vi "MAVLink Packet Sequence.vi"(7 "FGV Method":T1, 11 "Packet Sequence In":u8) -> (3 "Packet Sequence Out":u8)   [LabVIEW 2014]
uses:
  Controls/FGV Methods.ctl
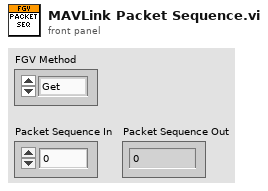
[diagram p1: front panel]
types:
  T1 = typedef "FGV Methods.ctl" = enum16{"Get", "Set"}
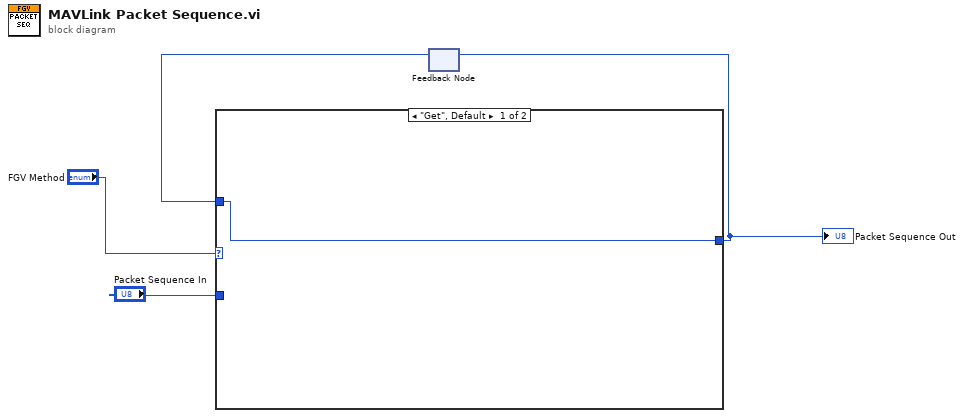
[diagram p0: block diagram]
diagram:
  n1 = feedback #1() -> (w3:u8)  [unwired: 1 in]
  n2 = case shown="\"Get\", Default" "FGV Method" {
    tunnel: "Packet Sequence In" -> [_ w6]
    tunnel: [w5 w6] -> w1
    tunnel: w3 -> [w5 _]
    frame "Get", Default {
    }
    frame "Set" {
    }
  }
  "Packet Sequence Out" <- w1
  n3 = feedback-in #1(w1) -> ()
